vi "Read.vi"(11 "ChannelValue in":refnum<class "DoubleChannelValue.lvclass">) -> (2 "Channel":refnum<class "Channel.lvclass">)   [LabVIEW 2020, in "Vecto.lvlib" / "DoubleChannelValue.lvclass"]
uses:
  DoubleChannelValue.lvclass
  Channel/Channel.lvclass
  DoubleChannelValue.lvclass/DoubleChannelValue.ctl
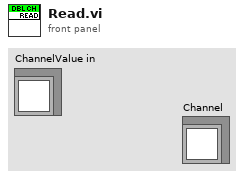
[diagram p1: front panel]
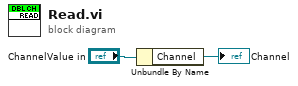
[diagram p0: block diagram]
diagram:
  n1 = Unbundle By Name("ChannelValue in") -> ("Channel"=→"Channel":refnum<class "Channel.lvclass">)
